vi "2_Hot_Films_12_1_00.vi"() -> (5 "Plug in titles":string[](array[string]), 7 "Plug in values":string[](array[string]))   [LabVIEW 2010]
uses:
  Controls/Post_Process.ctl
  Globals/Meas_global.vi
  Globals/Plug_in_data_global.vi
  <vilib>/Analysis/3filter.llb/Butterworth Filter (DBL).vi
  <vilib>/Analysis/NI_AALBase.lvlib
  <vilib>/Analysis/NI_AALPro.lvlib
panel:
  in  "Case Constant\n(See Context Help)":bool
  out "Max Correlation":dbl format="%.2f"
  in  "Approx Delay":dbl=23.0 format="%.2f"
  out "XY Graph":cluster{dbl[], dbl[]}[](graph)
  out "Hot Film mean":dbl format="%.2f"
  out "ADV mean":dbl format="%.2f"
  in  "Approx period":dbl=80.0 format="%.2f"
  in  "End chop":i32=200
  in  "Start chop":i32=2000
  out "Auto End Chop":i32
  out "Product":dbl[][](graph)
  out "Hot Film":dbl[][](graph)
  out "ADV":dbl[][](graph)
  out "Trailing Auto correlation":cluster{dbl, dbl, dbl[]}[](graph)
  out "Correlation Coefficient":T1(graph)
  out "Clipped length":i32
  out "Auto Start Chop":i32
  out "U components":cluster{dbl[], dbl[]}[](graph)
  # "End chop"
  # "End chop"
  # "End chop"
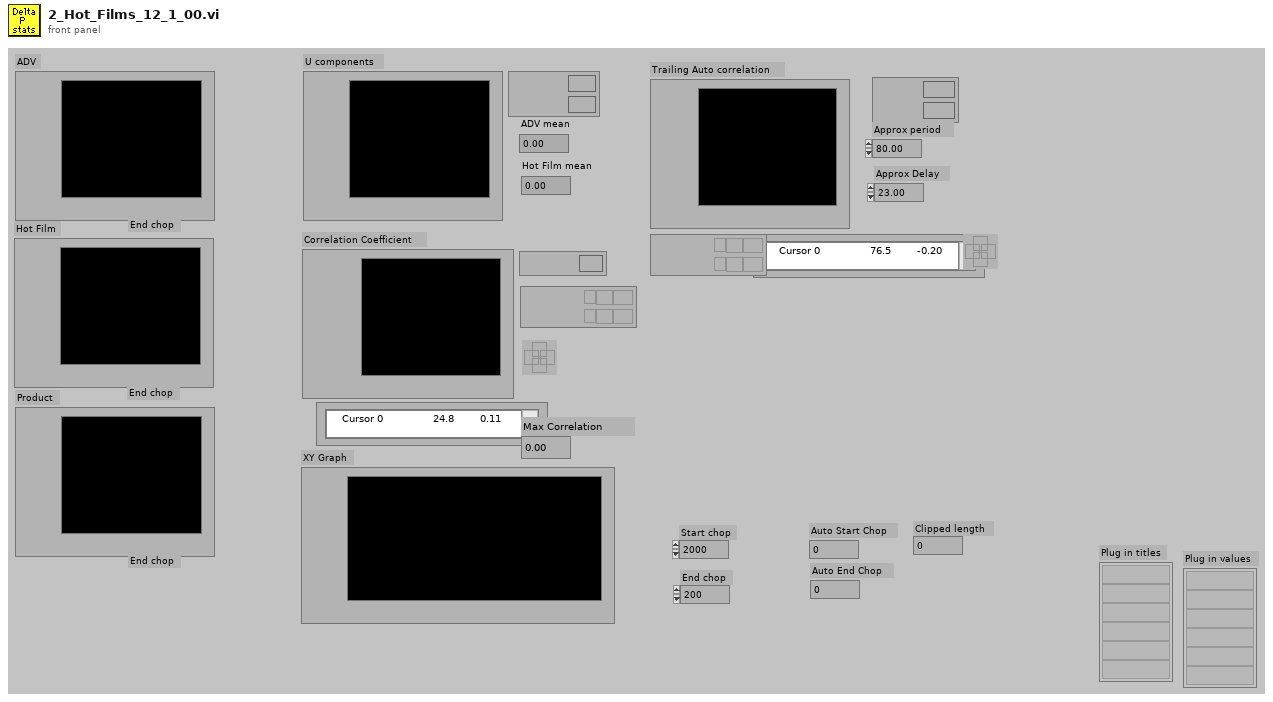
[diagram p1: front panel]
types:
  T1 = cluster{"Time":dbl[], "Correlation Coefficient":dbl[]}
  T2 = enum32{"Lowpass", "Highpass", "Bandpass", "Bandstop"}
  T3 = typedef "Post_Process.ctl" = enum16{"Take New Data", "Post Process Raw Data File"}
  T4 = typedef "Analysis_info_cluster.ctl" = cluster{"Colour":u32, "Inst type":T5, "Inst name":string, "Symbol":string, "Code name":string, "Extra Info":string, "Inst Array":T6, "Index":i32, "Voltage Index":i32, "Extra Titles":string[], "Extra Values":string[]}
  T5 = typedef "Inst_type.ctl" = enum16{"Propeller anemometer", "Raw voltage", "Pressure Transducer", "Pitot-static tube", "Preston tube", "Hot wire", "Cross wire 1", "Cross wire 2", "Generic Linear", "Generic Polynomial", "Generic BackPoly", "Fast FID", "Thermocouple", "Cold wire", "Pulsed Wire", "LDA Vel", "LDA Tran time", "LDA Arr time"}
  T6 = typedef "Instrument_Array.ctl" = enum16{"PWA", "LDA", "Analogue"}
  T7 = cluster{"Name":string, "X":dbl, "Y":dbl, "Z":dbl}[]
  T8 = cluster{"Name":string, "X":dbl, "Y":dbl, "Z":dbl}
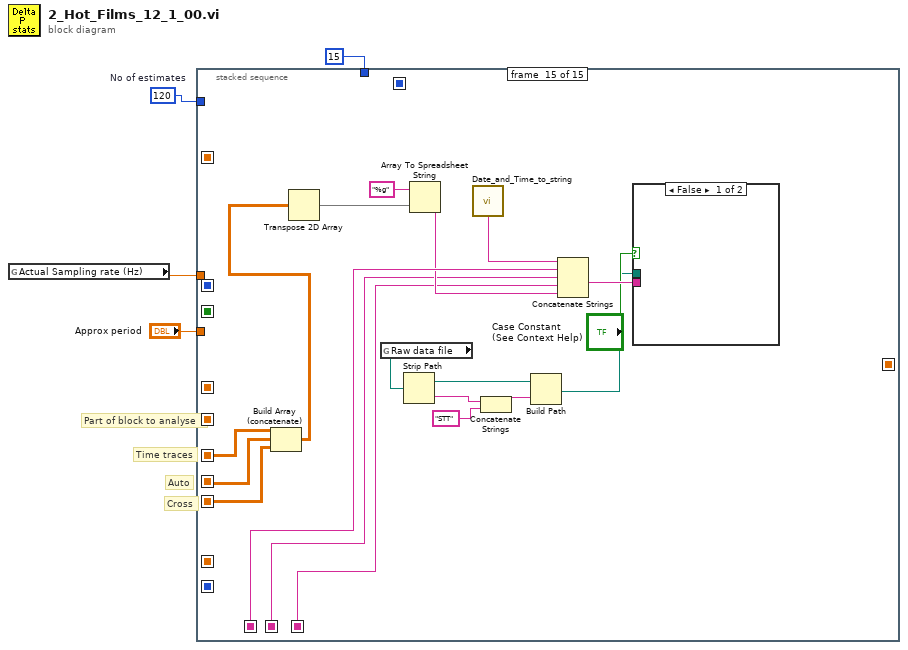
[diagram p0: block diagram]
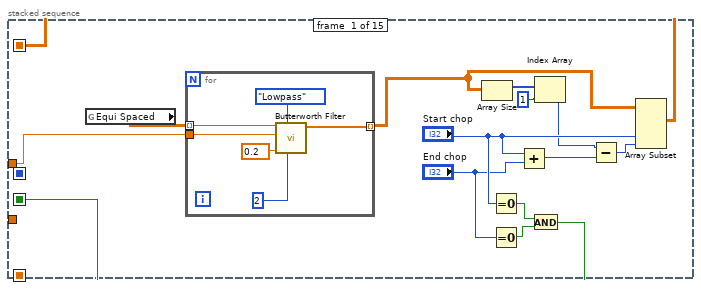
[diagram p2: hidden frame]
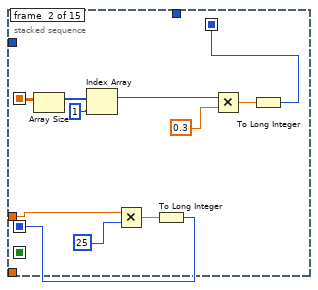
[diagram p3: hidden frame]
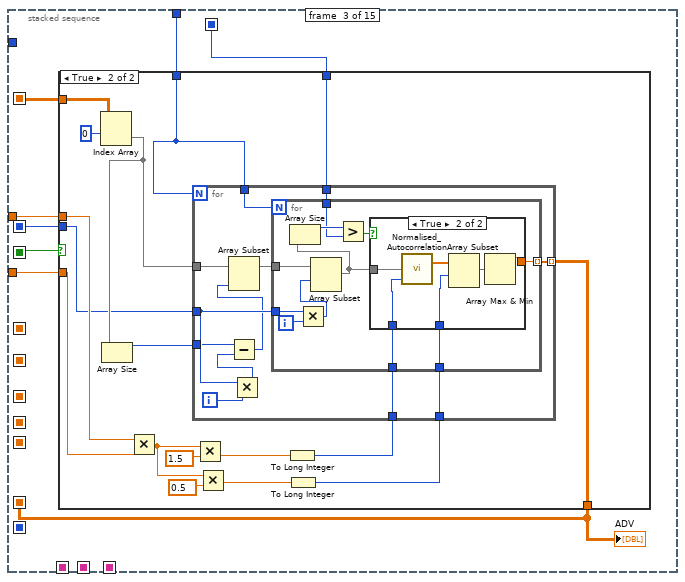
[diagram p4: hidden frame]
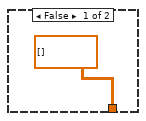
[diagram p5: hidden frame]
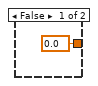
[diagram p6: hidden frame]
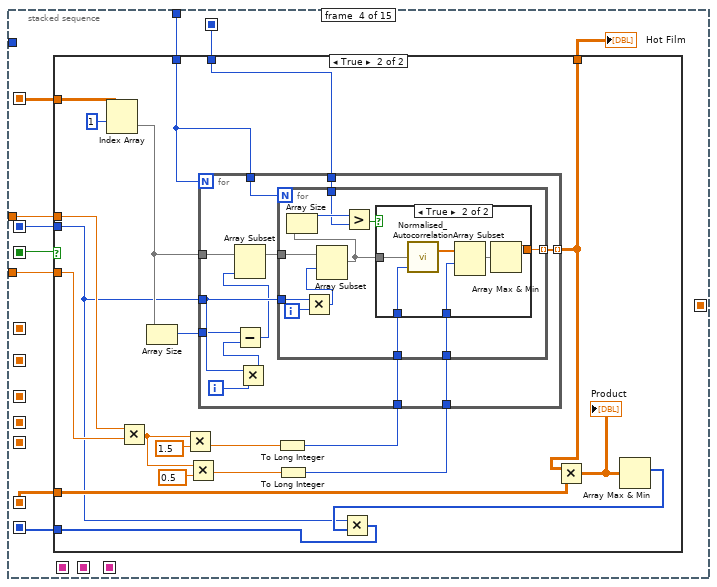
[diagram p7: hidden frame]
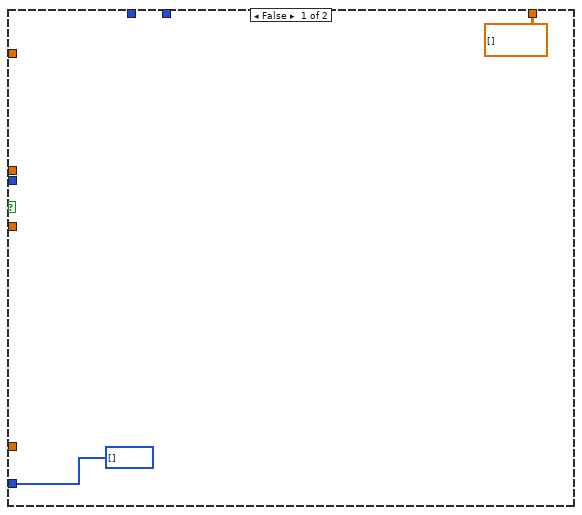
[diagram p8: hidden frame]
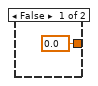
[diagram p9: hidden frame]
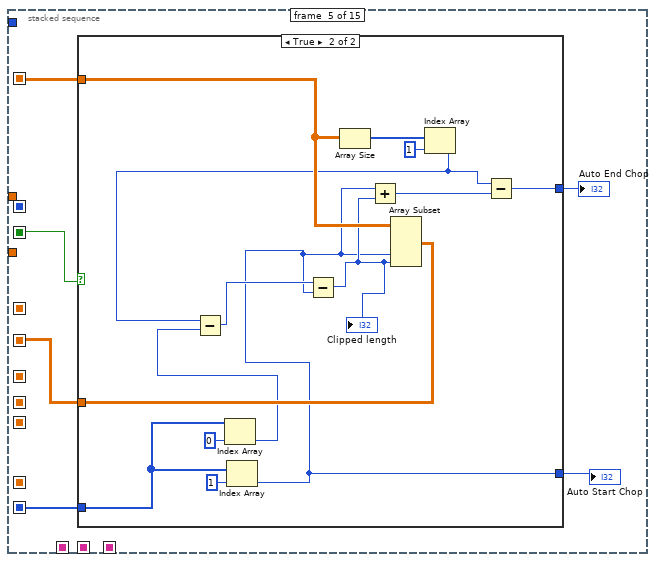
[diagram p10: hidden frame]
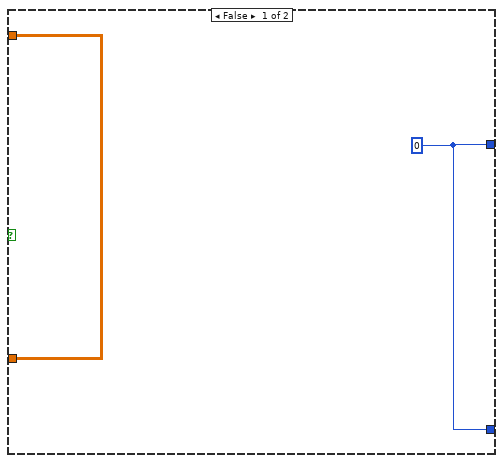
[diagram p11: hidden frame]
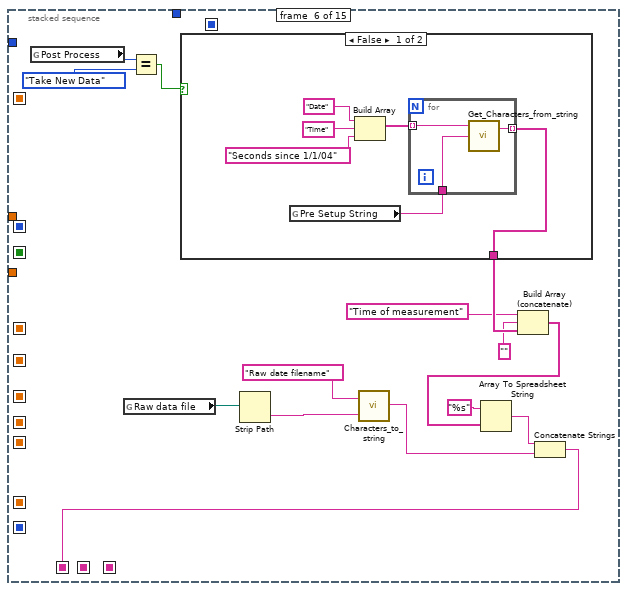
[diagram p12: hidden frame]
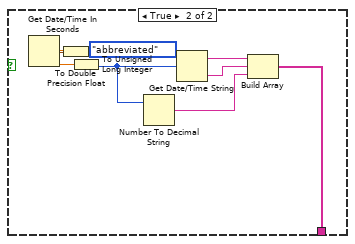
[diagram p13: hidden frame]
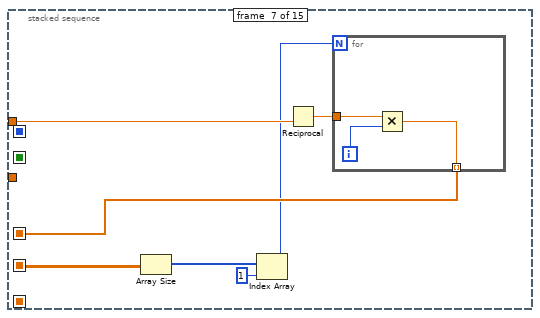
[diagram p14: hidden frame]
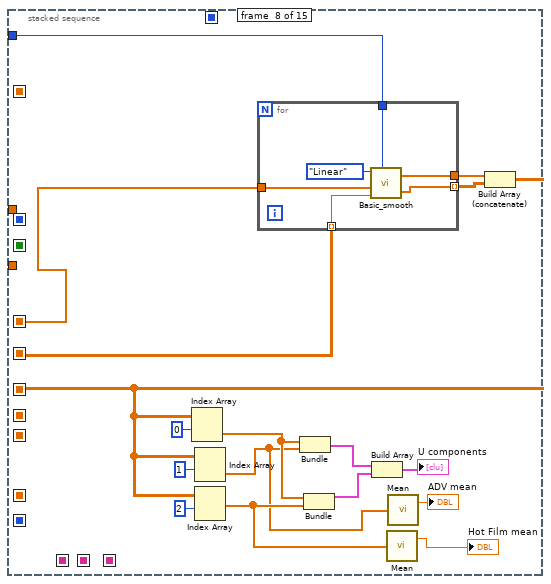
[diagram p15: hidden frame]
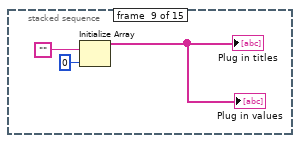
[diagram p16: hidden frame]
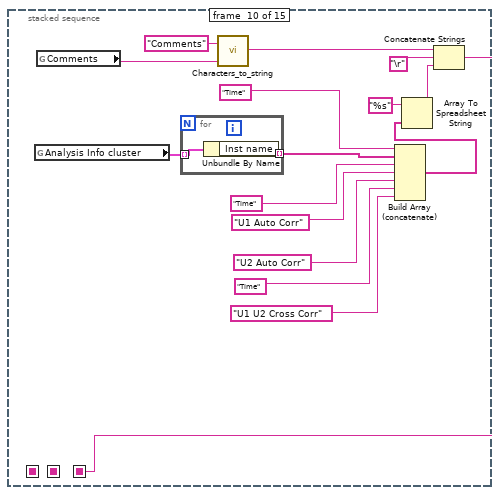
[diagram p17: hidden frame]
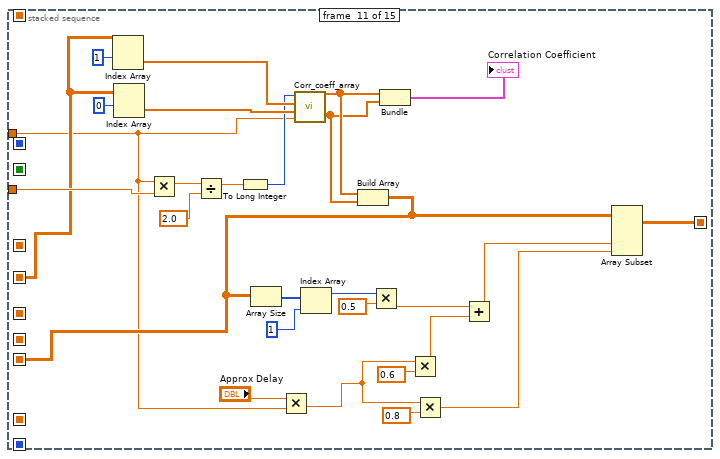
[diagram p18: hidden frame]
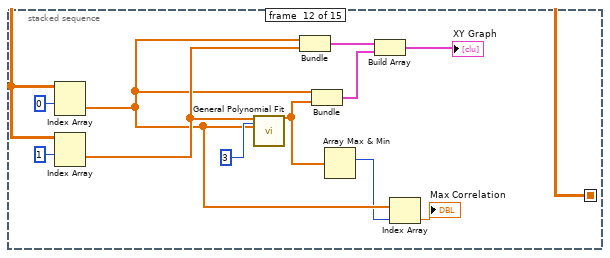
[diagram p19: hidden frame]
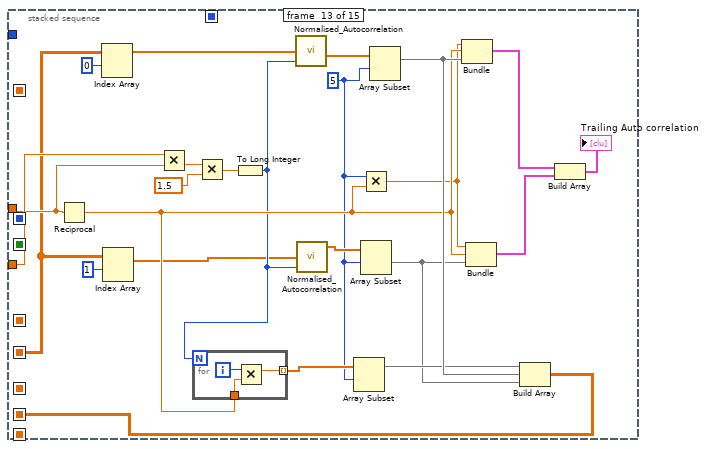
[diagram p20: hidden frame]
diagram:
  w4 = 120  # No of estimates
  # "Cross"
  # "Auto"
  # "Part of block to analyse"
  # "Time traces"
  n1 = global read "Meas_global.vi" "Actual Sampling rate (Hz)"() -> (w1:dbl)
  n2 = stacked-sequence {
    seq-local: [_ _ _ _ _ _ _ _ _ w255 _ _ _ _ _] -> [_ _ _ _ _ _ _ _ _ _ _ _ _ _ w356]
    seq-local: [_ _ _ _ _ _ w213 _ _ _ _ _ _ _ _] -> [_ _ _ _ _ _ _ w234 _ _ _ _ _ _ _]
    seq-local: [_ _ _ _ _ _ _ w226 _ _ _ _ _ _ _] -> [_ _ _ _ _ _ _ _ _ _ _ _ _ _ w362]
    seq-local: [_ _ _ _ _ w183 _ _ _ _ _ _ _ _ _] -> [_ _ _ _ _ _ _ _ _ _ _ _ _ _ w366]
    seq-local: [_ _ _ _ w160 _ _ _ _ _ _ _ _ _ _] -> [_ _ _ _ _ _ w209 w230 _ _ w282 _ w309 _ _]
    seq-local: [_ _ _ _ _ _ _ _ _ _ _ _ w322 _ _] -> [_ _ _ _ _ _ _ _ _ _ _ _ _ _ w361]
    seq-local: [_ _ _ _ _ _ _ _ _ _ w276 _ _ _ _] -> [_ _ _ _ _ _ _ _ _ _ _ _ _ _ w360]
    seq-local: [_ _ w38 _ _ _ _ _ _ _ _ _ _ _ _] -> [_ _ _ w101 _ _ _ _ _ _ _ _ _ _ _]
    seq-local: [_ _ _ w100 _ _ _ _ _ _ _ _ _ _ _] -> [_ _ _ _ w159 _ _ _ _ _ _ _ _ _ _]
    seq-local: [_ _ _ _ _ _ _ _ _ _ _ _ _ w334 _] -> [_ _ _ _ _ _ _ _ _ _ _ _ _ _ w355]
    seq-local: [_ w27 _ _ _ _ _ _ _ _ _ _ _ _ _] -> [_ _ w43 w99 _ _ _ _ _ _ _ _ _ _ _]
    seq-local: [_ w26 _ _ _ _ _ _ _ _ _ _ _ _ _] -> [_ _ w39 w95 _ _ _ _ _ _ _ _ _ _ _]
    seq-local: [_ _ _ _ _ _ _ _ _ _ w275 _ _ _ _] -> [_ _ _ _ _ _ _ _ _ _ _ w299 _ _ _]
    seq-local: [w8 _ _ _ _ _ _ _ _ _ _ _ _ _ _] -> [_ w25 w36 w92 w156 _ _ _ _ _ _ _ _ _ _]
    seq-local: [w9 _ _ _ _ _ _ _ _ _ _ _ _ _ _] -> [_ _ w37 w93 w155 _ _ _ _ _ _ _ _ _ _]
    tunnel: w1 -> [w6 w29 w41 w97 _ _ w212 _ _ _ w273 _ w320 _ _]
    tunnel: w4 -> [_ _ _ _ _ _ _ w231 _ _ _ _ _ _ _]
    tunnel: "Approx period" -> [_ _ w42 w98 _ _ _ _ _ _ w283 _ w321 _ _]
    tunnel: 15 -> [_ _ w40 w96 _ _ _ _ _ _ _ _ _ _ _]
    frame #0 {
      n3 = global read "Plug_in_data_global.vi" "Equi Spaced"() -> (w7:dbl[][])
      n4 = for {
        tunnel: [w21] -> w5 mode=indexing
        tunnel: w6 -> [w20]
        tunnel: w7 -> [w19] mode=indexing
        n5 = call-poly <vilib>:"Butterworth Filter.vi"("order"=2, "filter type"=T2."Lowpass", "low cutoff freq: fl"=0.2, "sampling freq: fs"=w20, "X"=w19) -> ("Filtered X"=w21:dbl[])  [unwired: 3 in, 1 out]
      }
      n6 = Array Size(array=w5) -> (size(s)=w11:i32[])
      n7 = Equal To 0?(x="Start chop") -> (x = 0?=w18:bool)
      n8 = Equal To 0?(x="End chop") -> (x = 0?=w17:bool)
      n9 = Add(x="Start chop", y="End chop") -> (x+y=w13:i32)
      n10 = And(x=w18, y=w17) -> (x .and. y?=w9:bool)
      n11 = Index Array(array=w11, index=1) -> (element=w12:i32)
      n12 = Subtract(x=w12, y=w13) -> (x-y=w14:i32)
      n13 = Array Subset(array=w5, index (col)="Start chop", length (col)=w14) -> (w8:dbl[][])  [unwired: 2 in]
    }
    frame #1 {
      n14 = Array Size(array=w25) -> (size(s)=w31:i32[])
      n15 = Index Array(array=w31, index=1) -> (element=w28:i32)
      n16 = Multiply(x=w29, y=25) -> (x*y=w34:dbl)
      n17 = To Long Integer(number=w34) -> (32bit integer=w26:i32)
      n18 = Multiply(x=w28, y=0.3) -> (x*y=w33:dbl)
      n19 = To Long Integer(number=w33) -> (32bit integer=w27:i32)
    }
    frame #2 {
      n20 = case shown="True" w37 {
        tunnel: w36 -> [_ w60]
        tunnel: [dbl[][] [] w57] -> w38
        tunnel: w43 -> [_ w56]
        tunnel: w42 -> [_ w48]
        tunnel: w41 -> [_ w47]
        tunnel: w40 -> [_ w46]
        tunnel: w39 -> [_ w45]
        frame False {
        }
        frame True {
          n21 = Index Array(array=w60, index (row)=0) -> (element=w59:dbl[])  [unwired: 1 in]
          n22 = Array Size(array=w59) -> (size(s)=w58:i32)
          n23 = Multiply(x=w47, y=w48) -> (x*y=w52:dbl)
          n24 = Multiply(x=w52, y=1.5) -> (x*y=w54:dbl)
          n25 = Multiply(x=w52, y=0.5) -> (x*y=w51:dbl)
          n26 = To Long Integer(number=w54) -> (32bit integer=w50:i32)
          n27 = To Long Integer(number=w51) -> (32bit integer=w49:i32)
          n28 = for {
            N: w46 -> [_]
            tunnel: w45 -> [w71]
            tunnel: w59 -> [w67]
            tunnel: w46 -> [w73]
            tunnel: w58 -> [w70]
            tunnel: [w65] -> w57 mode=indexing
            tunnel: w56 -> [w64]
            tunnel: w50 -> [w63]
            tunnel: w49 -> [w62]
            i -> [w72]
            n29 = Multiply(x=w71, y=w72) -> (x*y=w69:i32)
            n30 = Subtract(x=w70, y=w69) -> (x-y=w68:i32)
            n31 = Array Subset(array=w67, length=w68) -> (w66:dbl[])  [unwired: 1 in]
            n32 = for {
              N: w73 -> [_]
              tunnel: w71 -> [w82]
              tunnel: w66 -> [w81]
              tunnel: [w80] -> w65 mode=indexing
              tunnel: w64 -> [w76]
              tunnel: w63 -> [w75]
              tunnel: w62 -> [w74]
              i -> [w84]
              n33 = Multiply(x=w82, y=w84) -> (x*y=w83:i32)
              n34 = Array Subset(array=w81, index=w83) -> (w79:dbl[])  [unwired: 1 in]
              n35 = Array Size(array=w79) -> (size(s)=w77:i32)
              n36 = Greater?(x=w77, y=w76) -> (0:w78:bool)
              n37 = case shown="True" w78 {
                tunnel: [0.0 w91] -> w80
                tunnel: w79 -> [_ w88]
                tunnel: w75 -> [_ w87]
                tunnel: w74 -> [_ w86]
                frame False {
                }
                frame True {
                  n38 = call "Normalised_Autocorrelation.vi"("Autocorrelation length"=w87, "Array"=w88) -> ("Normalised Auto corr"=w90:dbl[])  [unwired: 1 in]
                  n39 = Array Subset(array=w90, index=w86) -> (w89:dbl[])  [unwired: 1 in]
                  n40 = Array Max & Min(array=w89) -> (max value=w91:dbl)  [unwired: 3 out]
                }
              }
            }
          }
        }
      }
      "ADV" <- w38
    }
    frame #3 {
      n41 = case shown="True" w93 {
        tunnel: w92 -> [_ w123]
        tunnel: w101 -> [_ w122]
        tunnel: [i32[] [] w119] -> w100
        tunnel: w99 -> [_ w116]
        tunnel: w98 -> [_ w113]
        tunnel: w97 -> [_ w112]
        tunnel: w96 -> [_ w106]
        tunnel: w95 -> [_ w105]
        tunnel: [dbl[][] [] w104] -> w94
        frame False {
        }
        frame True {
          n42 = Index Array(array=w123, index (row)=1) -> (element=w118:dbl[])  [unwired: 1 in]
          n43 = Multiply(x=w112, y=w113) -> (x*y=w109:dbl)
          n44 = Array Size(array=w118) -> (size(s)=w117:i32)
          n45 = Multiply(x=w109, y=1.5) -> (x*y=w114:dbl)
          n46 = Multiply(x=w109, y=0.5) -> (x*y=w108:dbl)
          n47 = To Long Integer(number=w114) -> (32bit integer=w111:i32)
          n48 = To Long Integer(number=w108) -> (32bit integer=w107:i32)
          n49 = for {
            N: w106 -> [_]
            tunnel: w105 -> [w134]
            tunnel: w118 -> [w130]
            tunnel: w106 -> [w136]
            tunnel: w117 -> [w133]
            tunnel: [w128] -> w104 mode=indexing
            tunnel: w116 -> [w127]
            tunnel: w111 -> [w126]
            tunnel: w107 -> [w125]
            i -> [w135]
            n50 = Multiply(x=w134, y=w135) -> (x*y=w132:i32)
            n51 = Subtract(x=w133, y=w132) -> (x-y=w131:i32)
            n52 = Array Subset(array=w130, length=w131) -> (w129:dbl[])  [unwired: 1 in]
            n53 = for {
              N: w136 -> [_]
              tunnel: w134 -> [w145]
              tunnel: w129 -> [w144]
              tunnel: [w143] -> w128 mode=indexing
              tunnel: w127 -> [w139]
              tunnel: w126 -> [w138]
              tunnel: w125 -> [w137]
              i -> [w147]
              n54 = Multiply(x=w145, y=w147) -> (x*y=w146:i32)
              n55 = Array Subset(array=w144, index=w146) -> (w142:dbl[])  [unwired: 1 in]
              n56 = Array Size(array=w142) -> (size(s)=w140:i32)
              n57 = Greater?(x=w140, y=w139) -> (0:w141:bool)
              n58 = case shown="True" w141 {
                tunnel: [0.0 w154] -> w143
                tunnel: w142 -> [_ w151]
                tunnel: w138 -> [_ w150]
                tunnel: w137 -> [_ w149]
                frame False {
                }
                frame True {
                  n59 = call "Normalised_Autocorrelation.vi"("Autocorrelation length"=w150, "Array"=w151) -> ("Normalised Auto corr"=w153:dbl[])  [unwired: 1 in]
                  n60 = Array Subset(array=w153, index=w149) -> (w152:dbl[])  [unwired: 1 in]
                  n61 = Array Max & Min(array=w152) -> (max value=w154:dbl)  [unwired: 3 out]
                }
              }
            }
          }
          n62 = Multiply(x=w104, y=w122) -> (x*y=w121:dbl[][])
          "Product" <- w121
          n63 = Array Max & Min(array=w121) -> (max index (indices)=w120:i32[])  [unwired: 3 out]
          n64 = Multiply(x=w105, y=w120) -> (x*y=w119:i32[])
        }
      }
      "Hot Film" <- w94
    }
    frame #4 {
      n65 = case shown="True" w155 {
        tunnel: [w162 w176] -> w160
        tunnel: w156 -> [w162 w175]
        tunnel: w159 -> [_ w169]
        tunnel: [w161 w164] -> w158
        tunnel: [w161 w163] -> w157
        frame False {
          w161 = 0
        }
        frame True {
          n66 = Index Array(array=w169, index=0) -> (element=w171:i32)
          n67 = Index Array(array=w169, index=1) -> (element=w163:i32)
          n68 = Array Size(array=w175) -> (size(s)=w173:i32[])
          n69 = Index Array(array=w173, index=1) -> (element=w166:i32)
          n70 = Subtract(x=w166, y=w171) -> (x-y=w168:i32)
          n71 = Subtract(x=w168, y=w163) -> (x-y=w167:i32)
          "Clipped length" <- w167
          n72 = Add(x=w163, y=w167) -> (x+y=w165:i32)
          n73 = Array Subset(array=w175, index (col)=w163, length (col)=w167) -> (w176:dbl[][])  [unwired: 2 in]
          n74 = Subtract(x=w166, y=w165) -> (x-y=w164:i32)
        }
      }
      "Auto End Chop" <- w158
      "Auto Start Chop" <- w157
    }
    frame #5 {
      n75 = global read "Meas_global.vi" "Post Process"() -> (w189:T3)
      n76 = global read "Meas_global.vi" "Raw data file"() -> (w178:path)
      n77 = Equal?(x=w189, y=Post_Process."Take New Data" ("Post Process")) -> (x = y?=w188:bool)
      n78 = case shown="False" w188 {
        tunnel: [w191 w201] -> w182
        frame False {
          n79 = global read "Meas_global.vi" "Pre Setup String"() -> (w192:string)
          n80 = Build Array("Date", "Time", "Seconds since 1/1/04") -> (w193:string[])
          n81 = for {
            tunnel: w193 -> [w199] mode=indexing
            tunnel: w192 -> [w198]
            tunnel: [w197] -> w191 mode=indexing
            n82 = call "Get_Characters_from_string.vi"("Input string"=w198, "Variable name"=w199) -> ("Value"=w197:string)  [unwired: 1 in, 1 out]
          }
        }
        frame True {
          n83 = Get Date/Time In Seconds() -> (seconds since 1Jan1904=w200:timestamp)
          n84 = To Double Precision Float(number=w200) -> (double precision float=w204:dbl)
          n85 = To Unsigned Long Integer(number=w204) -> (unsigned 32bit integer=w203:u32)
          n86 = Number To Decimal String(number=w203) -> (decimal integer string=w202:string)  [unwired: 1 in]
          n87 = Get Date/Time String(date format (0)=enum16{"short", "long", "abbreviated"}."abbreviated", seconds (now)=w203) -> (date string=w206:string, time string=w205:string)  [unwired: 1 in]
          n88 = Build Array(w206, w205, w202) -> (w201:string[])
        }
      }
      n89 = Strip Path(path=w178) -> (name=w177:string)  [unwired: 1 out]
      n90 = call "Characters_to_string.vi"("Characters to write"=w177, "Label for characters"="Raw date filename") -> ("Output string"=w184:string)
      n91 = Build Array (concatenate)("Time of measurement", "" ("Value"), w182) -> (w179:string[])
      n92 = Array To Spreadsheet String(array=w179, 3:"%s" ("format string")) -> (spreadsheet string=w185:string)  [unwired: 1 in]
      n93 = Concatenate Strings(w185, w184) -> (w183:string)
    }
    frame #6 {
      n94 = Array Size(array=w209) -> (size(s)=w210:i32[])
      n95 = Index Array(array=w210, index=1) -> (element=w208:i32)
      n96 = Reciprocal(x=w212) -> (1/x=w214:dbl)
      n97 = for {
        N: w208 -> [_]
        tunnel: w214 -> [w217]
        tunnel: [w215] -> w213 mode=indexing
        i -> [w216]
        n98 = Multiply(x=w217, y=w216) -> (x*y=w215:dbl)
      }
    }
    frame #7 {
      n99 = for {
        tunnel: w234 -> [w239]
        tunnel: w230 -> [w238] mode=indexing
        tunnel: [w237] -> w233
        tunnel: [w236] -> w232 mode=indexing
        tunnel: w231 -> [w235]
        n100 = call "Basic_smooth.vi"("Smoothing"=enum16{"Linear", "Logarithmic"}."Linear", "X array in"=w239, "Y array in"=w238, "No of estimates output"=w235) -> ("X array Out"=w237:dbl[], "Y array Out"=w236:dbl[])  [unwired: 1 in]
      }
      n101 = Build Array (concatenate)(w233, w232) -> (w226:dbl[][])
      n102 = Index Array(array=w226, index (row)=0) -> (element=w225:dbl[])  [unwired: 1 in]
      n103 = Index Array(array=w226, index (row)=1) -> (element=w220:dbl[])  [unwired: 1 in]
      n104 = Index Array(array=w226, index (row)=2) -> (element=w221:dbl[])  [unwired: 1 in]
      n105 = Bundle(w225, w220) -> (w224:cluster{dbl[], dbl[]})  [unwired: 1 in]
      n106 = Bundle(w225, w221) -> (w223:cluster{dbl[], dbl[]})  [unwired: 1 in]
      n107 = Build Array(w224, w223) -> (→"U components":cluster{dbl[], dbl[]}[])
      n108 = call <vilib>:"Mean.vi"("X"=w221) -> ("mean"=→"Hot Film mean":dbl)  [unwired: 1 out]
      n109 = call <vilib>:"Mean.vi"("X"=w220) -> ("mean"=→"ADV mean":dbl)  [unwired: 1 out]
    }
    frame #8 {
      n110 = Initialize Array("", 0) -> (→"Plug in titles" →"Plug in values":string[])
    }
    frame #9 {
      n111 = global read "Meas_global.vi" "Analysis Info cluster"() -> (w254:T4[])
      n112 = global read "Meas_global.vi" "Comments"() -> (w259:string)
      n113 = for {
        tunnel: w254 -> [w261] mode=indexing
        tunnel: [w260] -> w247 mode=indexing
        n114 = Unbundle By Name(w261) -> ("Inst name"=w260:string)
      }
      n115 = call "Characters_to_string.vi"("Characters to write"=w259, "Label for characters"="Comments") -> ("Output string"=w257:string)
      n116 = Build Array (concatenate)("Time", w247, "Time", "U1 Auto Corr", "U2 Auto Corr", "Time", "U1 U2 Cross Corr") -> (w250:string[])
      n117 = Array To Spreadsheet String(array=w250, 3:"%s" ("format string")) -> (spreadsheet string=w249:string)  [unwired: 1 in]
      n118 = Concatenate Strings(w257, "\r", w249) -> (w255:string)
    }
    frame #10 {
      n119 = Index Array(array=w282, index (row)=1) -> (element=w289:dbl[])  [unwired: 1 in]
      n120 = Index Array(array=w282, index (row)=0) -> (element=w288:dbl[])  [unwired: 1 in]
      n121 = Multiply(x=w273, y=w283) -> (x*y=w265:dbl)
      n122 = Divide(x=w265, y=2.0) -> (x/y=w263:dbl)
      n123 = To Long Integer(number=w263) -> (32bit integer=w281:i32)
      n124 = Multiply(x="Approx Delay", y=w273) -> (x*y=w262:dbl)
      n125 = call "Corr_coeff_array.vi"("Sampling frequency"=w273, "U2"=w288, "U1"=w289, "Slippage range"=w281) -> ("Correlation Coefficient"=w280:dbl[], "Time"=w285:dbl[])
      n126 = Build Array(w285, w280) -> (w276:dbl[][])
      n127 = Array Size(array=w276) -> (size(s)=w279:i32[])
      n128 = Index Array(array=w279, index=1 ("Index")) -> (element=w272:i32)
      n129 = Multiply(x=w272, y=0.5) -> (x*y=w269:dbl)
      n130 = Bundle("Time"=w285, "Correlation Coefficient"=w280) -> (→"Correlation Coefficient":T1)  [unwired: 1 in]
      n131 = Multiply(x=w262, y=0.6) -> (x*y=w270:dbl)
      n132 = Multiply(x=w262, y=0.8) -> (x*y=w266:dbl)
      n133 = Add(x=w269, y=w270) -> (x+y=w268:dbl)
      n134 = Array Subset(array=w276, index (col)=w268, length (col)=w266) -> (w275:dbl[][])  [unwired: 2 in]
    }
    frame #11 {
      n135 = Index Array(array=w299, index (row)=0 ("Index")) -> (element=w292:dbl[])  [unwired: 1 in]
      n136 = Index Array(array=w299, index (row)=1 ("Index")) -> (element=w296:dbl[])  [unwired: 1 in]
      n137 = call <vilib>:"General Polynomial Fit.vi"("Y"=w296, "polynomial order"=3, "X"=w292) -> ("Best Polynomial Fit"=w293:dbl[])  [unwired: 9 in, 3 out]
      n138 = Bundle(w292, w296) -> (w298:cluster{dbl[], dbl[]})  [unwired: 1 in]
      n139 = Bundle(w292, "Best Polynomial Fit"=w293) -> (w295:cluster{dbl[], "Best Polynomial Fit":dbl[]})  [unwired: 1 in]
      n140 = Array Max & Min(array=w293) -> (max index (indices)=w291:i32)  [unwired: 3 out]
      n141 = Build Array(w298, w295) -> (→"XY Graph":cluster{dbl[], "Best Polynomial Fit":dbl[]}[])
      n142 = Index Array(array=w292, index=w291) -> (element=→"Max Correlation":dbl)
    }
    frame #12 {
      w308 = 5
      n143 = Reciprocal(x=w320) -> (1/x=w311:dbl)
      n144 = Index Array(array=w309, index (row)=0) -> (element=w324:dbl[])  [unwired: 1 in]
      n145 = Index Array(array=w309, index (row)=1) -> (element=w306:dbl[])  [unwired: 1 in]
      n146 = Multiply(x=w321, y=w320) -> (x*y=w319:dbl)
      n147 = Multiply(x=w319, y=1.5) -> (x*y=w317:dbl)
      n148 = To Long Integer(number=w317) -> (32bit integer=w307:i32)
      n149 = for {
        N: w307 -> [_]
        tunnel: w311 -> [w327]
        tunnel: [w326] -> w313 mode=indexing
        i -> [w328]
        n150 = Multiply(x=w328, y=w327) -> (x*y=w326:dbl)
      }
      n151 = call "Normalised_Autocorrelation.vi"("Autocorrelation length"=w307, "Array"=w324) -> ("Normalised Auto corr"=w316:dbl[])  [unwired: 1 in]
      n152 = call "Normalised_Autocorrelation.vi"("Autocorrelation length"=w307, "Array"=w306) -> ("Normalised Auto corr"=w315:dbl[])  [unwired: 1 in]
      n153 = Array Subset(array=w313, index=w308) -> (w312:dbl[])  [unwired: 1 in]
      n154 = Multiply(x=w308, y=w311) -> (x*y=w310:dbl)
      n155 = Array Subset(array=w315, index=w308) -> (w305:dbl[])  [unwired: 1 in]
      n156 = Array Subset(array=w316, index=w308) -> (w314:dbl[])  [unwired: 1 in]
      n157 = Bundle(w310, w311, w314) -> (w303:cluster{dbl, dbl, dbl[]})  [unwired: 1 in]
      n158 = Bundle(w310, w311, w305) -> (w304:cluster{dbl, dbl, dbl[]})  [unwired: 1 in]
      n159 = Build Array(w312, w314, w305) -> (w322:dbl[][])
      n160 = Build Array(w303, w304) -> (→"Trailing Auto correlation":cluster{dbl, dbl, dbl[]}[])
    }
    frame #13 {
      n161 = global read "Meas_global.vi" "Position"() -> (w346:T7)
      n162 = Index Array(array=w346, index=0) -> (element=w345:T8)
      n163 = Index Array(array=w346, index=3) -> (element=w344:T8)
      n164 = Unbundle By Name(w345) -> ("Name"=w331:string, "X"=w342:dbl, "Y"=w341:dbl, "Z"=w340:dbl)
      n165 = Unbundle By Name(w344) -> ("Name"=w329:string, "X"=w339:dbl, "Y"=w338:dbl, "Z"=w337:dbl)
      n166 = Concatenate Strings(w331, " " ("Output string")) -> (w343:string)
      n167 = Concatenate Strings(w329, " " ("Output string")) -> (w333:string)
      n168 = call "XYZ_Pos_to_string.vi"("Position label"=w343, "Z"=w340, "Y"=w341, "X"=w342) -> ("Output string"=w336:string)
      n169 = call "XYZ_Pos_to_string.vi"("Position label"=w333, "Z"=w337, "Y"=w338, "X"=w339) -> ("Output string"=w335:string)
      n170 = Concatenate Strings(w336, w335) -> (w334:string)
    }
    frame #14 {
      n171 = Build Array (concatenate)(w362, w361, w360) -> (w358:dbl[][])
      n172 = Transpose 2D Array(2D array=w358) -> (transposed array=w367:dbl[][])
      n173 = global read "Meas_global.vi" "Raw data file"() -> (w353:path)
      n174 = Strip Path(path=w353) -> (stripped path=w350:path, name=w352:string)
      n175 = Array To Spreadsheet String(array=w367, 3:"%g" ("format string")) -> (spreadsheet string=w357:string)  [unwired: 1 in]
      n176 = call "Date_and_Time_to_string.vi"() -> ("Date and time (spreadsheet)"=w359:string)
      n177 = Concatenate Strings(w352, "STT") -> (w351:string)
      n178 = Build Path(base path=w350, name or relative path=w351) -> (appended path=w349:path)
      n179 = Concatenate Strings(w359, w366, w355, w356, w357) -> (w364:string)
      n180 = case shown="False" "Case Constant\n(See Context Help)" {
        tunnel: w364 -> [_ w370]
        tunnel: w349 -> [_ w369]
        frame False {
        }
        frame True {
          w368 = FALSE  # advisory dialog? (display:T)
          n181 = call "Write_Characters_To_File.vi"("file path (dialog if empty)"=w369, "advisory dialog? (display:T)"=w368, "character string"=w370) -> ()  [unwired: 5 in, 1 out]
        }
      }
    }
  }
